vi "PCUseClassData.vi"() -> ()   [LabVIEW 2014]
uses:
  MsgWithClassDataTypedef.ctl
  Data/Data.lvclass
panel:
  in  "ButtonB":bool
  in  "ButtonA":bool
  out "NowTime":timestamp
  out "MsgString":string
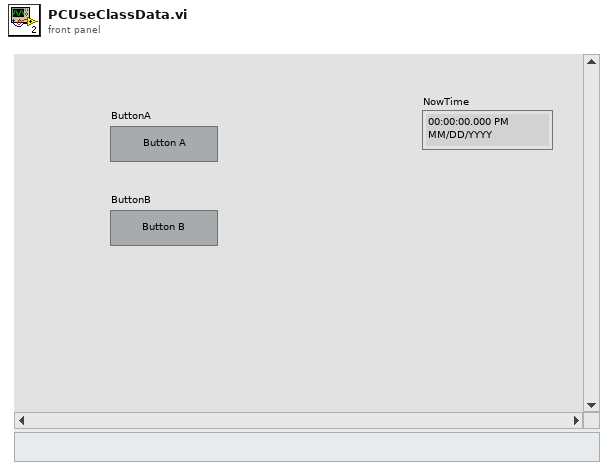
[diagram p1: front panel]
types:
  T1 = typedef "MsgWithClassDataTypedef.ctl" = cluster{"CMD":string, "DataClass":refnum<class "Data.lvclass">}
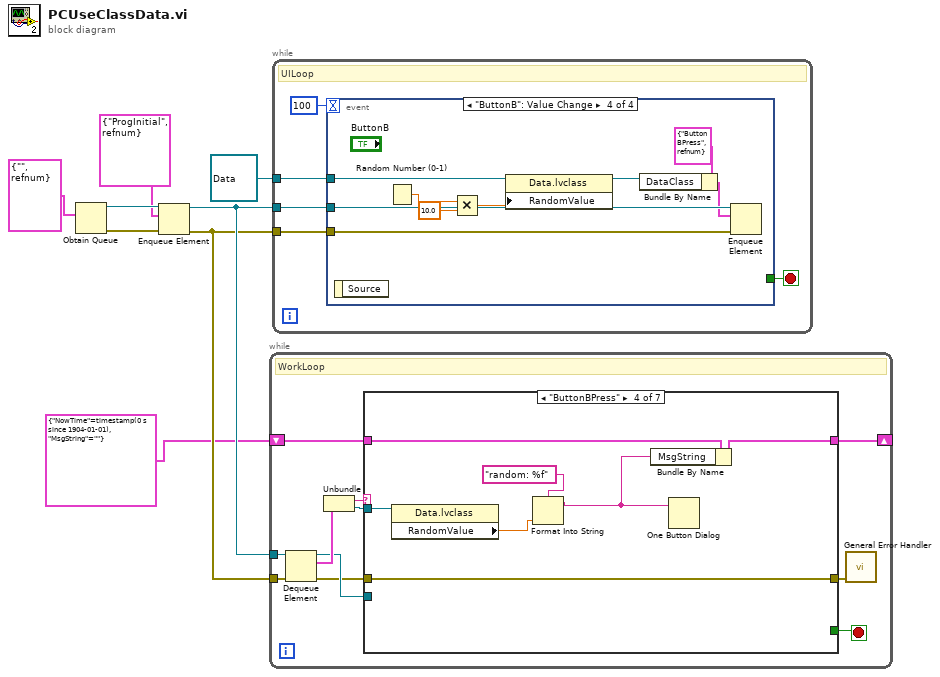
[diagram p0: block diagram]
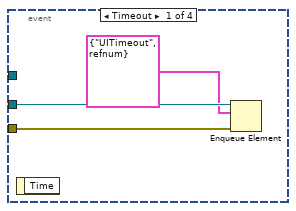
[diagram p2: hidden frame]
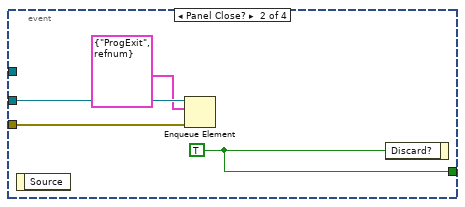
[diagram p3: hidden frame]
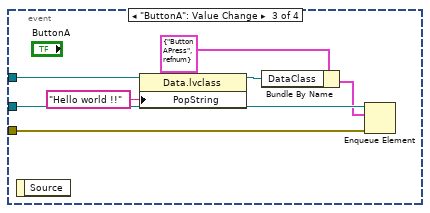
[diagram p4: hidden frame]
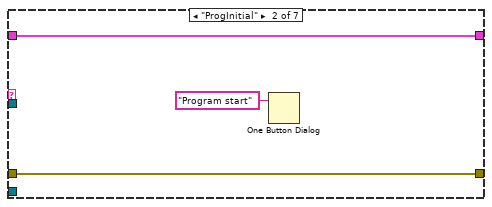
[diagram p6: hidden frame]
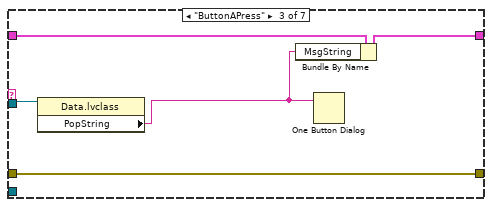
[diagram p7: hidden frame]
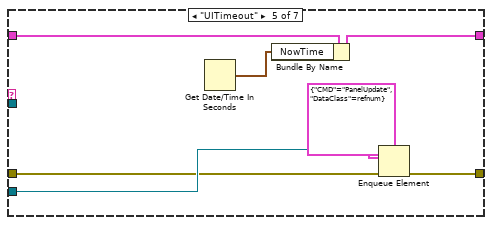
[diagram p8: hidden frame]
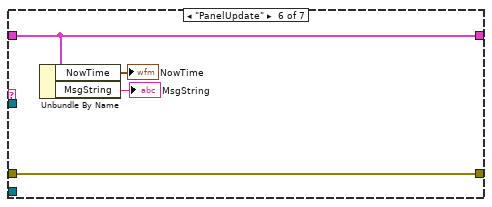
[diagram p9: hidden frame]
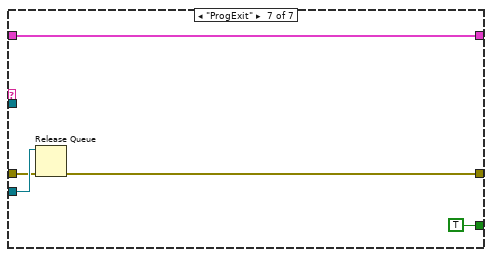
[diagram p10: hidden frame]
diagram:
  n1 = Obtain Queue(element data type=T1 {"CMD"="", "DataClass"=refnum}) -> (queue out=w8:refnum<queue>, error out=w7:errorcluster)  [unwired: 4 in, 1 out]
  n2 = Enqueue Element(queue=w8, element=T1 {"CMD"="ProgInitial", "DataClass"=refnum}, error in (no error)=w7) -> (queue out=w6:refnum<queue>, error out=w5:errorcluster)  [unwired: 1 in, 1 out]
  n3 = while {
    tunnel: w6 -> [w19]
    tunnel: w5 -> [w18]
    shift-right: [w16] -> _
    shift-left: cluster{"NowTime":timestamp, "MsgString":string} {"NowTime"=timestamp(0 s since 1904-01-01), "MsgString"=""} -> [w15]
    stop <- w12 stop-if-true
    # "WorkLoop"
    n4 = Dequeue Element(queue=w19, error in (no error)=w18) -> (queue out=w14:refnum<queue>, element=w17:T1, error out=w13:errorcluster)  [unwired: 1 in, 1 out]
    n5 = Unbundle(w17) -> ("CMD"=w11:string, "DataClass"=w10:refnum<class "Data.lvclass">)
    n6 = case shown="\"ButtonBPress\"" w11 {
      tunnel: [w21 w23 w28 w35 w42 w47 w52] -> w16
      tunnel: w15 -> [w21 w23 w29 w36 w43 w47 w52]
      tunnel: w14 -> [_ _ _ _ w40 _ w51]
      tunnel: w13 -> [w20 w22 w27 w32 w39 w44 w50]
      tunnel: [_ _ _ _ _ _ TRUE ("Discard?")] -> w12
      tunnel: w10 -> [_ _ w26 w31 _ _ _]
      tunnel: [w20 w22 w27 w32 w37 w44 w48] -> w9
      frame Default {
      }
      frame "ProgInitial" {
        n7 = One Button Dialog(message="Program start") -> ()  [unwired: 1 in, 1 out]
      }
      frame "ButtonAPress" {
        n8 = property class="Data.lvclass"(reference=w26) -> ("PopString"=w25:string)  [unwired: 1 in, 2 out]
        n9 = Bundle By Name(cluster=w29, "MsgString"=w25) -> (w28:cluster{"NowTime":timestamp, "MsgString":string})
        n10 = One Button Dialog(message=w25) -> ()  [unwired: 1 in, 1 out]
      }
      frame "ButtonBPress" {
        n11 = property class="Data.lvclass"(reference=w31) -> ("RandomValue"=w30:dbl)  [unwired: 1 in, 2 out]
        n12 = Format Into String(format string="random: %f", w30) -> (resulting string=w33:string)  [unwired: 2 in, 1 out]
        n13 = Bundle By Name(cluster=w36, "MsgString"=w33) -> (w35:cluster{"NowTime":timestamp, "MsgString":string})
        n14 = One Button Dialog(message=w33) -> ()  [unwired: 1 in, 1 out]
      }
      frame "UITimeout" {
        n15 = Get Date/Time In Seconds() -> (seconds since 1Jan1904=w41:timestamp)
        n16 = Bundle By Name(cluster=w43, "NowTime"=w41) -> (w42:cluster{"NowTime":timestamp, "MsgString":string})
        n17 = Enqueue Element(queue=w40, element=T1 {"CMD"="PanelUpdate", "DataClass"=refnum}, error in (no error)=w39) -> (error out=w37:errorcluster)  [unwired: 1 in, 2 out]
      }
      frame "PanelUpdate" {
        n18 = Unbundle By Name(w47) -> ("NowTime"=→"NowTime":timestamp, "MsgString"=→"MsgString":string)
      }
      frame "ProgExit" {
        n19 = Release Queue(queue=w51, error in (no error)=w50) -> (error out=w48:errorcluster)  [unwired: 1 in, 2 out]
      }
    }
    n20 = call <vilib>:"General Error Handler.vi"("error in (no error)"=w9) -> ()  [unwired: 10 in, 5 out]
  }
  n21 = while {
    tunnel: w6 -> [w56]
    tunnel: w5 -> [w55]
    tunnel: refnum<class "Data.lvclass"> refnum ("DataClass") -> [w53]
    stop <- w54 stop-if-true
    # "UILoop"
    n22 = event shown="[3] \"ButtonB\": Value Change" {
      selector: _ -> [_ _ _ _]
      dyn-events: _ -> [_ _ _ _]
      timeout: 100 -> [_ _ _ _]
      tunnel: w56 -> [w60 w64 w71 w80]
      tunnel: w55 -> [w59 w63 w70 w79]
      tunnel: [_ w62 _ _] -> w54
      tunnel: w53 -> [_ _ w67 w76]
      event Timeout {
        n23 = event-data() -> ()  [unwired: 1 in, 1 out]
        n24 = Enqueue Element(queue=w60, element=T1 {"CMD"="UITimeout", "DataClass"=refnum}, error in (no error)=w59) -> ()  [unwired: 1 in, 3 out]
      }
      event Panel Close? {
        w62 = TRUE ("Discard?")
        n25 = event-data() -> ()  [unwired: 1 in, 1 out]
        n26 = Enqueue Element(queue=w64, element=T1 {"CMD"="ProgExit", "DataClass"=refnum}, error in (no error)=w63) -> ()  [unwired: 1 in, 3 out]
        n27 = event-data("Discard?"=w62) -> ()  [unwired: 1 in, 1 out]
      }
      event "ButtonA": Value Change {
        n28 = event-data() -> ()  [unwired: 1 in, 1 out]
        n29 = property class="Data.lvclass"(reference=w67, "PopString"="Hello world !!") -> (reference out=w66:refnum<class "Data.lvclass">)  [unwired: 1 in, 1 out]
        n30 = Bundle By Name(cluster=T1 {"CMD"="ButtonAPress", "DataClass"=refnum}, "DataClass"=w66) -> (w68:T1)
        n31 = Enqueue Element(queue=w71, element=w68, error in (no error)=w70) -> ()  [unwired: 1 in, 3 out]
      }
      event "ButtonB": Value Change {
        n32 = event-data() -> ()  [unwired: 1 in, 1 out]
        n33 = Random Number (0-1)() -> (number: 0 to 1=w74:dbl)
        n34 = Multiply(x=w74, y=10.0) -> (x*y=w73:dbl)
        n35 = property class="Data.lvclass"(reference=w76, "RandomValue"=w73) -> (reference out=w75:refnum<class "Data.lvclass">)  [unwired: 1 in, 1 out]
        n36 = Bundle By Name(cluster=T1 {"CMD"="ButtonBPress", "DataClass"=refnum}, "DataClass"=w75) -> (w77:T1)
        n37 = Enqueue Element(queue=w80, element=w77, error in (no error)=w79) -> ()  [unwired: 1 in, 3 out]
      }
    }
  }
